vi "Write ErrorOrSuccess JSON.vi"(8 "error in (no error)":errorcluster, 10 "wamplv.lvlib:ErrorOrSuccess JSON.lvclass":refnum<class "ErrorOrSuccess JSON.lvclass">, 11 "SubscribeResult JSON in":refnum<class "SubscribeResult JSON.lvclass">) -> (0 "error out":errorcluster, 3 "SubscribeResult JSON out":refnum<class "SubscribeResult JSON.lvclass">)   [LabVIEW 2020, in "wamplv.lvlib" / "SubscribeResult JSON.lvclass"]
uses:
  SubscribeResult JSON.lvclass
  SubscribeResult JSON.lvclass/SubscribeResult JSON.ctl
  Private/Message loop classes/ErrorOrSuccess JSON/ErrorOrSuccess JSON.lvclass
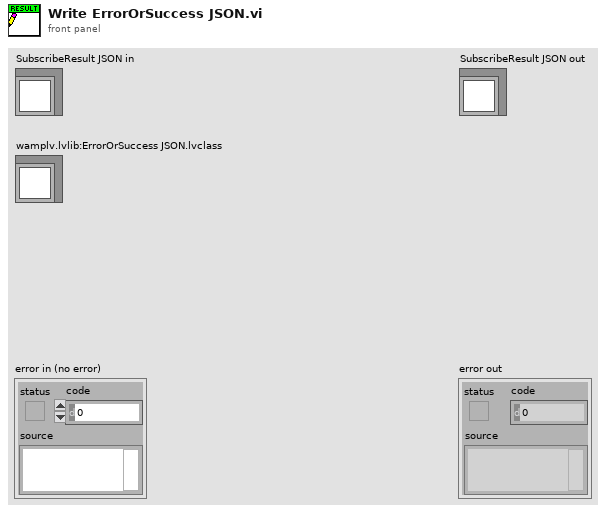
[diagram p1: front panel]
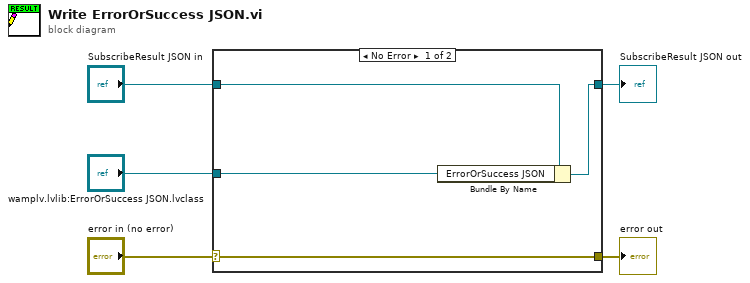
[diagram p0: block diagram]
diagram:
  n1 = case shown="No Error" "error in (no error)" {
    selector: "error in (no error)" -> [w9 w10]
    tunnel: [w9 w10] -> w4
    tunnel: [w7 w11] -> w2
    tunnel: "SubscribeResult JSON in" -> [w8 w11]
    tunnel: "wamplv.lvlib:ErrorOrSuccess JSON.lvclass" -> [w6 _]
    frame No Error {
      n2 = Bundle By Name(cluster=w8, "ErrorOrSuccess JSON"=w6) -> (w7:refnum<class "SubscribeResult JSON.lvclass">)
    }
    frame Error {
    }
  }
  "error out" <- w4
  "SubscribeResult JSON out" <- w2
